vi "python simple example numeric.vi"() -> ()   [LabVIEW 2018]
panel:
  out "return value":i32[](array[numeric])
  in  "Python version":string="3.8"
  in  "function name":string="print_func"
  in  "module path":path=path "C:/Users/tony_/Downloads/2020_04_24_PNG_HDF5_Benchmark_Tony/2020_04_24_PNG_HDF5_Benchmark_Tony/testmodule.py"
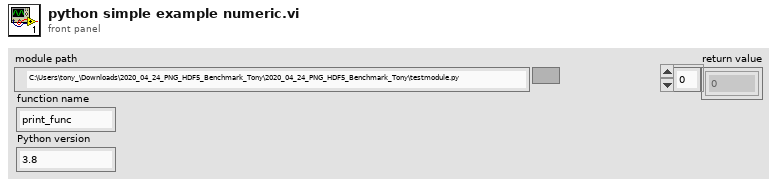
[diagram p1: front panel]
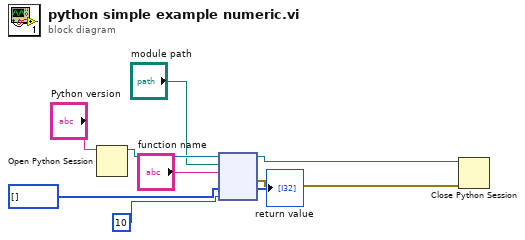
[diagram p0: block diagram]
diagram:
  n1 = Open Python Session(python version="Python version") -> (session out=w8:refnum<k35>)  [unwired: 2 in, 1 out]
  n2 = node(w8, "module path", "function name", i32[] [], 10) -> (w7:refnum<k35>, w6:errorcluster, →"return value":i32[])  [unwired: 2 in, 2 out]
  n3 = Close Python Session(session in=w7, error in=w6) -> ()  [unwired: 1 out]
